vi "PLC_comm.vi"() -> ()   [LabVIEW 2017]
uses:
  <vilib>/DATA AHEAD/SP7/typedefs/PLC Type.ctl
  <vilib>/Utility/error.llb/DialogType.ctl
  <vilib>/addons/database/Connection.llb/DB Tools Open Connec (String).vi
  Global/Global 1.vi
  Global/DATA LOG.vi
  <vilib>/DATA AHEAD/SP7/functions/write/write Dint array.vi
  <vilib>/DATA AHEAD/SP7/functions/write/writeString.vi
  <vilib>/DATA AHEAD/SP7/functions/read/read Dint array.vi
  <vilib>/DATA AHEAD/SP7/functions/read/read real array.vi
  <vilib>/DATA AHEAD/SP7/functions/read/read String.vi
  <vilib>/addons/database/NI_Database_API.lvlib
  <vilib>/DATA AHEAD/SP7/SP7.lvlib
panel:
  out "IP1 7":string
  out "PLC 7":bool
  out "IP1 6":string
  out "PLC 6":bool
  out "IP1 5":string
  out "PLC 5":bool
  out "PLC 4":bool
  out "PLC 3":bool
  out "PLC 2":bool
  out "PLC 1":bool
  out "IP1 4":string
  out "IP1 3":string
  out "IP1 2":string
  out "IP1":string
  in  "stop":bool
  out "error out":errorcluster
  in  "error in (no error)":errorcluster
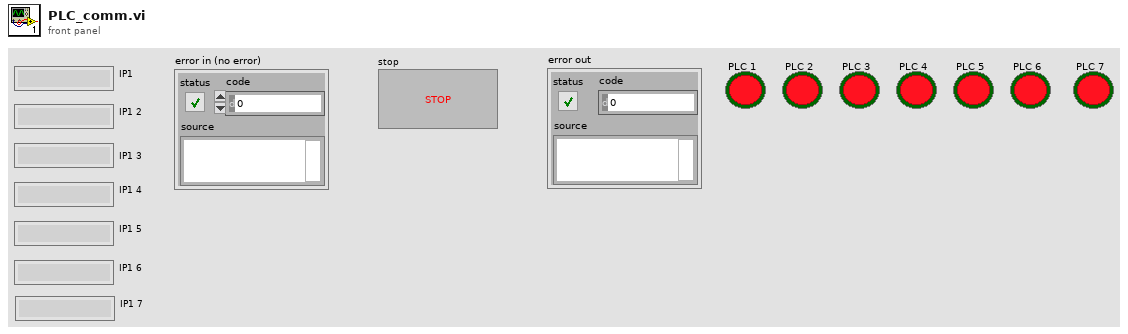
[diagram p1: front panel]
types:
  T1 = typedef "DialogType.ctl" = u16
  T2 = typedef "SP7.lvlib/PLC Type.ctl" = enum16{"S7 200", "S7 300/400", "S7 1200", "S7 1500", "LOGO!8"}
  T3 = typedef "NI_Database_API.lvlib/Conn ObjectReference.ctl" = refnum<k1>
  T4 = typedef "SP7.lvlib/S7 Connection.ctl" = cluster{"TCP Connection Ref":refnum<k5>, "IP address":string, "timeout ms":i32, "Connected?":bool, "PLC Type":T2, "Rack S7 400":u8, "Slot S7 400":u8, "PDU Size":u16, "connection semaphore":T5}
  T5 = typedef "Semaphore RefNum" = refnum<k1>
diagram:
  w2 = T1 0 items=["no dialog", "OK message", "continue or stop message", "OK message + warnings", "continue/stop + warnings"]  # type of dialog (OK msg:1)
  w4 = i32[] [0, 0, 0, 0, 0]  # I/P
  w5 = i32[] [0, 0]  # Input
  w7 = i32[] [0, 0]  # Input
  w8 = i32[] [0, 0]  # Input
  w10 = i32[] [0, 0]  # Input
  w6 = i32[] [0, 0, 0, 0, 0]  # I/P
  w9 = i32[] [0, 0, 0, 0, 0]  # I/P
  w11 = i32[] [0, 0, 0, 0, 0]  # I/P
  w12 = i32[] [0, 0, 0, 0, 0]  # I/P
  w13 = i32[] [0, 0]  # Input
  w14 = i32[] [0, 0]  # Input
  w15 = i32[] [0, 0, 0, 0, 0]  # I/P
  w16 = i32[] [0, 0, 0, 0, 0]  # I/P
  w17 = i32[] [0, 0]  # Input
  w18 = i32[] [0, 0]  # I/P
  w19 = i32[] [0, 0]  # Input
  # "OP 80"
  # "OP 70"
  # "OP 60"
  # "OP 50"
  # "OP 40"
  # "OP 30"
  # "OP 20"
  # "OP 10"
  n1 = call "path_db.vi"("error in"="error in (no error)") -> ("error out"=w171:errorcluster, "resulting string"=w176:string)  [unwired: 9 in]
  n2 = call-poly <vilib>:"DB Tools Open Connection.vi"("error in (no error)"=w171, "connection information"=w176) -> ("error out"=w175:errorcluster, "connection reference"=w174:T3)  [unwired: 6 in]
  n3 = call <vilib>:"DB Tools Select Data.vi"("error in (no error)"=w175, "columns"=string[] ["PLC_IP_1", "PLC_IP_2", "PLC_IP_3", "PLC_IP_4", "PLC_IP_5", "PLC_IP_6", "PLC_IP_7"], "table"="IP_SETTING", "connection reference"=w174) -> ("error out"=w173:errorcluster, "data"=w172:variant[][])  [unwired: 2 in, 1 out]
  n4 = call "PADMINI_varient_to_data.vi"("error in (no error)"=w173, "data"=w172) -> ("error out"=w26:errorcluster, "Array"=w167:string[][])  [unwired: 8 in]
  n5 = call "PADMINI_AUTO_CYCLE STATE.vi"("Enum"=enum16{"Read", "Write"}."Write", "error in (no error)"=w26, "Input"=w19) -> ("error out"=w153:errorcluster)  [unwired: 7 in, 1 out]
  n6 = Index Array(array=w167, index (row)=0) -> (element=w166:string[])  [unwired: 1 in]
  n7 = call "PADMINI_AUTO_BARCODE_STRING.vi"("Enum"=enum16{"Read", "Write"}."Write", "error in (no error)"=w153, "Input"=string[] ["", ""]) -> ("error out"=w150:errorcluster)  [unwired: 7 in, 1 out]
  n8 = call "PADMINI_AUTO_BARCODE_STATUS.vi"("Enum"=enum16{"Read", "Write"}."Write", "error in (no error)"=w150, "I/P"=w18) -> ("error out"=w148:errorcluster)  [unwired: 7 in, 1 out]
  n9 = call "PADMINI_AUTO_CYCLE VALUE 10.vi"("Enum"=enum16{"Read", "Write"}."Write", "error in (no error)"=w148, "Input"=dbl[] [0.0]) -> ("error out"=w142:errorcluster)  [unwired: 7 in, 1 out]
  n10 = call "PADMINI_AUTO_CYCLE STATE 20.vi"("Enum"=enum16{"Read", "Write"}."Write", "error in (no error)"=w142, "Input"=w5) -> ("error out"=w140:errorcluster)  [unwired: 7 in, 1 out]
  n11 = call "PADMINI_AUTO_CYCLE VALUE 20.vi"("Enum"=enum16{"Read", "Write"}."Write", "error in (no error)"=w140, "Input"=dbl[] [0.0, 0.0, 0.0, 0.0]) -> ("error out"=w136:errorcluster)  [unwired: 7 in, 1 out]
  n12 = call "PADMINI_AUTO_BARCODE_STRING2.vi"("Enum"=enum16{"Read", "Write"}."Write", "error in (no error)"=w136, "Input"=string[] ["", "", "", "", "", "", ""]) -> ("error out"=w134:errorcluster)  [unwired: 7 in, 1 out]
  n13 = call "PADMINI_AUTO_BARCODE_STATUS 20.vi"("Enum"=enum16{"Read", "Write"}."Write", "error in (no error)"=w134, "I/P"=w4) -> ("error out"=w128:errorcluster)  [unwired: 7 in, 1 out]
  n14 = call "PADMINI_AUTO_BARCODE_STATUS 30.vi"("Enum"=enum16{"Read", "Write"}."Write", "error in (no error)"=w128, "I/P"=w6) -> ("error out"=w125:errorcluster)  [unwired: 7 in, 1 out]
  n15 = call "PADMINI_AUTO_CYCLE STATE 30.vi"("Enum"=enum16{"Read", "Write"}."Write", "error in (no error)"=w125, "Input"=w7) -> ("error out"=w124:errorcluster)  [unwired: 7 in, 1 out]
  n16 = call "PADMINI_AUTO_CYCLE VALUE 30.vi"("Enum"=enum16{"Read", "Write"}."Write", "error in (no error)"=w124, "Input"=dbl[] [0.0, 0.0]) -> ("error out"=w121:errorcluster)  [unwired: 7 in, 1 out]
  n17 = call "PADMINI_AUTO_BARCODE_STRING 30.vi"("Enum"=enum16{"Read", "Write"}."Write", "error in (no error)"=w121, "Input"=string[] ["", "", ""]) -> ("error out"=w100:errorcluster)  [unwired: 7 in, 1 out]
  n18 = call "PADMINI_AUTO_BARCODE_STATUS 40.vi"("Enum"=enum16{"Read", "Write"}."Write", "error in (no error)"=w100, "I/P"=w9) -> ("error out"=w99:errorcluster)  [unwired: 7 in, 1 out]
  n19 = call "PADMINI_AUTO_CYCLE VALUE 40.vi"("Enum"=enum16{"Read", "Write"}."Write", "error in (no error)"=w99, "Input"=dbl[] [0.0, 0.0, 0.0, 0.0]) -> ("error out"=w98:errorcluster)  [unwired: 7 in, 1 out]
  n20 = call "PADMINI_AUTO_CYCLE STATE 40.vi"("Enum"=enum16{"Read", "Write"}."Write", "error in (no error)"=w98, "Input"=w8) -> ("error out"=w97:errorcluster)  [unwired: 7 in, 1 out]
  n21 = call "PADMINI_AUTO_BARCODE_STATUS 50.vi"("Enum"=enum16{"Read", "Write"}."Write", "error in (no error)"=w97, "I/P"=w11) -> ("error out"=w82:errorcluster)  [unwired: 7 in, 1 out]
  n22 = call "PADMINI_AUTO_CYCLE STATE 50.vi"("Enum"=enum16{"Read", "Write"}."Write", "error in (no error)"=w82, "Input"=w10) -> ("error out"=w86:errorcluster)  [unwired: 7 in, 1 out]
  n23 = call "PADMINI_AUTO_CYCLE VALUE 50.vi"("Enum"=enum16{"Read", "Write"}."Write", "error in (no error)"=w86, "Input"=dbl[] [0.0, 0.0, 0.0]) -> ("error out"=w83:errorcluster)  [unwired: 7 in, 1 out]
  n24 = call "PADMINI_AUTO_BARCODE_STRING 50.vi"("Enum"=enum16{"Read", "Write"}."Write", "error in (no error)"=w83, "Input"=string[] ["", "", "", "", "", ""]) -> ("error out"=w59:errorcluster)  [unwired: 7 in, 1 out]
  n25 = call "PADMINI_AUTO_BARCODE_STATUS 60.vi"("Enum"=enum16{"Read", "Write"}."Write", "error in (no error)"=w59, "I/P"=w12) -> ("error out"=w63:errorcluster)  [unwired: 7 in, 1 out]
  n26 = call "PADMINI_AUTO_CYCLE STATE 60.vi"("Enum"=enum16{"Read", "Write"}."Write", "error in (no error)"=w63, "Input"=w13) -> ("error out"=w65:errorcluster)  [unwired: 7 in, 1 out]
  n27 = call "PADMINI_AUTO_CYCLE VALUE 60.vi"("Enum"=enum16{"Read", "Write"}."Write", "error in (no error)"=w65, "Input"=dbl[] [0.0, 0.0, 0.0, 0.0, 0.0]) -> ("error out"=w68:errorcluster)  [unwired: 7 in, 1 out]
  n28 = call "PADMINI_AUTO_BARCODE_STRING 60.vi"("Enum"=enum16{"Read", "Write"}."Write", "error in (no error)"=w68, "Input"=string[] ["", "", "", "", "", ""]) -> ("error out"=w35:errorcluster)  [unwired: 7 in, 1 out]
  n29 = call "PADMINI_AUTO_BARCODE_STATUS 70.vi"("Enum"=enum16{"Read", "Write"}."Write", "error in (no error)"=w35, "I/P"=w15) -> ("error out"=w38:errorcluster)  [unwired: 7 in, 1 out]
  n30 = call "PADMINI_AUTO_CYCLE STATE 70.vi"("Enum"=enum16{"Read", "Write"}."Read", "error in (no error)"=w38, "Input"=w14) -> ("error out"=w50:errorcluster)  [unwired: 7 in, 1 out]
  n31 = call "PADMINI_AUTO_CYCLE VALUE 70.vi"("Enum"=enum16{"Read", "Write"}."Write", "error in (no error)"=w50, "Input"=dbl[] [0.0, 0.0]) -> ("error out"=w47:errorcluster)  [unwired: 7 in, 1 out]
  n32 = call "PADMINI_AUTO_BARCODE_STRING 70.vi"("Enum"=enum16{"Read", "Write"}."Write", "error in (no error)"=w47, "Input"=string[] ["", ""]) -> ("error out"=w32:errorcluster)  [unwired: 7 in, 1 out]
  n33 = call "PADMINI_AUTO_BARCODE_STATUS 80.vi"("Enum"=enum16{"Read", "Write"}."Write", "error in (no error)"=w32, "I/P"=w16) -> ("error out"=w39:errorcluster)  [unwired: 7 in, 1 out]
  n34 = call "PADMINI_AUTO_CYCLE STATE 80.vi"("Enum"=enum16{"Read", "Write"}."Write", "error in (no error)"=w39, "Input"=w17) -> ("error out"=w43:errorcluster)  [unwired: 7 in, 1 out]
  n35 = call "PADMINI_AUTO_CYCLE VALUE 80.vi"("Enum"=enum16{"Read", "Write"}."Write", "error in (no error)"=w43, "Input"=sgl[] [0.0]) -> ("error out"=w46:errorcluster)  [unwired: 7 in, 1 out]
  n36 = call "PADMINI_AUTO_BARCODE_STRING 80.vi"("Enum"=enum16{"Read", "Write"}."Write", "error in (no error)"=w46, "Input"=string[] ["", "", ""]) -> ()  [unwired: 7 in, 2 out]
  n37 = Index Array(array=w166) -> (element #1=w115:string, element #2=w116:string, element #3=w110:string, element #4=w88:string, element #5=w71:string, element #6=w28:string, element #7=w27:string)  [unwired: 7 in]
  "IP1" <- w115
  "IP1 2" <- w116
  "IP1 3" <- w110
  "IP1 4" <- w88
  "IP1 5" <- w71
  "IP1 6" <- w28
  "IP1 7" <- w27
  n38 = call <vilib>:"connect.vi"("PLC Type"=PLC_Type."S7 1200" ("PLC Type 2"), "error in (no error)"=w26, "timeout [ms]"=1000 ("timeout [ms] 2"), "IP address"=w27) -> ("error out"=w29:errorcluster, "S7 Connection out"=w1:T4)  [unwired: 6 in]
  n39 = call <vilib>:"connect.vi"("PLC Type"=PLC_Type."S7 1200" ("PLC Type 2"), "error in (no error)"=w26, "timeout [ms]"=1000 ("timeout [ms] 2"), "IP address"=w71) -> ("error out"=w76:errorcluster, "S7 Connection out"=w75:T4)  [unwired: 6 in]
  n40 = call <vilib>:"connect.vi"("PLC Type"=PLC_Type."S7 1200" ("PLC Type 2"), "error in (no error)"=w26, "timeout [ms]"=1000 ("timeout [ms] 2"), "IP address"=w28) -> ("error out"=w56:errorcluster, "S7 Connection out"=w55:T4)  [unwired: 6 in]
  n41 = call <vilib>:"connect.vi"("PLC Type"=PLC_Type."S7 1200" ("PLC Type 2"), "error in (no error)"=w26, "timeout [ms]"=1000 ("timeout [ms] 2"), "IP address"=w88) -> ("error out"=w91:errorcluster, "S7 Connection out"=w92:T4)  [unwired: 6 in]
  n42 = call <vilib>:"connect.vi"("PLC Type"=PLC_Type."S7 1200" ("PLC Type 2"), "error in (no error)"=w26, "timeout [ms]"=1000 ("timeout [ms] 2"), "IP address"=w116) -> ("error out"=w131:errorcluster, "S7 Connection out"=w130:T4)  [unwired: 6 in]
  n43 = call <vilib>:"connect.vi"("PLC Type"=PLC_Type."S7 1200" ("PLC Type 2"), "error in (no error)"=w26, "timeout [ms]"=1000 ("timeout [ms] 2"), "IP address"=w110) -> ("error out"=w112:errorcluster, "S7 Connection out"=w111:T4)  [unwired: 6 in]
  n44 = call <vilib>:"connect.vi"("PLC Type"=PLC_Type."S7 1200" ("PLC Type 2"), "error in (no error)"=w26, "timeout [ms]"=1000, "IP address"=w115) -> ("error out"=w157:errorcluster, "S7 Connection out"=w156:T4)  [unwired: 6 in]
  n45 = while {
    shift-right: [w179] -> w23
    shift-left: w1 -> [w189]
    shift-right: [w187] -> w24
    shift-left: w29 -> [w188]
    tunnel: w27 -> [w178]
    stop <- w181 stop-if-true
    # "OP 90 - 100 - 110"
    n46 = flat-sequence {
      tunnel: [w265] -> w185
      tunnel: [w266] -> w180
      tunnel: w188 -> [w304]
      tunnel: w189 -> [w303]
      tunnel: w178 -> [w285]
      tunnel: [w285] -> w177
      tunnel: [w372] -> w187
      tunnel: [w371] -> w179
      tunnel: w185 -> [w374]
      tunnel: w180 -> [w373]
      tunnel: w177 -> [w370]
      frame #0 {
        w206 = u16 75 ("Data Block #")
        w231 = u16 72 ("Data Block #")
        w257 = u16 70 ("Data Block #")
        w215 = u16 71 ("Data Block #")
        w245 = u16 69 ("Data Block #")
        # "OP100 OK\nOP 100 NG"
        # "AUTO WRITE"
        n47 = global read "DATA LOG.vi" "OP 90 Outputs"() -> (w302:bool)
        n48 = case shown="True" w302 {
          tunnel: w303 -> [w355 w368]
          tunnel: [w356 w357] -> w262
          tunnel: [w355 w358] -> w263
          tunnel: w304 -> [w356 w365]
          frame False {
          }
          frame True {
            w369 = u16 70  # Data Block #
            n49 = call "PADMINI_AUTO_BARCODE_STATUS 90.vi"("Enum"=enum16{"Read", "Write"}."Read", "error in (no error)"=w365) -> ("error out"=w364:errorcluster, "O/P"=w366:i32[])  [unwired: 8 in]
            n50 = global write "DATA LOG.vi" "OP 90 Outputs"(FALSE) -> ()
            n51 = call-poly <vilib>:"write DB.vi"("DINT input array"=w366, "error in (no error)"=w364, "Data Block #"=w369, "S7 Connection in"=w368) -> ("error out"=w360:errorcluster, "S7 Connection out"=w359:T4)  [unwired: 4 in, 2 out]
            n52 = call-poly <vilib>:"write DB.vi"("DINT input array"=i32[] [0] ("Data Byte"), "error in (no error)"=w360, "Data Block #"=u16 69, "S7 Connection in"=w359) -> ("error out"=w357:errorcluster, "S7 Connection out"=w358:T4)  [unwired: 4 in, 2 out]
          }
        }
        n53 = global read "DATA LOG.vi" "OP 90 reset"() -> (w261:bool)
        n54 = case shown="True" w261 {
          tunnel: w262 -> [w330 w339]
          tunnel: [w330 w338] -> w250
          tunnel: w263 -> [w331 w337]
          tunnel: [w331 w336] -> w251
          frame False {
          }
          frame True {
            n55 = global write "DATA LOG.vi" "OP 90 reset"(FALSE) -> ()
            n56 = call-poly <vilib>:"write DB.vi"("Item offset [byte]"=u16 4 ("Data Block #"), "DINT input array"=i32[] [0], "error in (no error)"=w339, "Data Block #"=u16 69, "S7 Connection in"=w337) -> ("error out"=w338:errorcluster, "S7 Connection out"=w336:T4)  [unwired: 3 in, 2 out]
          }
        }
        n57 = global read "DATA LOG.vi" "Auto Cycle On"() -> (w197:bool)
        n58 = Boolean To (0,1)(Boolean=w197) -> (0, 1=w196:i16)
        n59 = Build Array(w196) -> (w195:i16[])
        n60 = global read "Global 1.vi" "Filtered BARCODE selected"() -> (w260:string[])
        n61 = call-poly <vilib>:"write DB.vi"("Item offset [byte]"=u32 20, "DINT input array"=w195, "error in (no error)"=w250, "Data Block #"=w257, "S7 Connection in"=w251) -> ("error out"=w255:errorcluster, "S7 Connection out"=w254:T4)  [unwired: 3 in, 2 out]
        n62 = call-poly <vilib>:"write DB.vi"("Item offset [byte]"=u32 24, "Input STRINGS"=w260, "error in (no error)"=w255, "String length reserved in DB (default=254)"=u16 15, "Data Block #"=w257, "S7 Connection in"=w254) -> ("error out"=w252:errorcluster, "S7 Connection out"=w253:T4)  [unwired: 2 in, 2 out]
        n63 = call-poly <vilib>:"read DB.vi"("error in (no error)"=w252, "items #"=u16 2 ("Items # [byte]"), "Data Block #"=w245, "S7 Connection in"=w253) -> ("error out"=w300:errorcluster, "DINT result array"=w298:i32[], "S7 Connection out"=w295:T4)  [unwired: 5 in]
        n64 = call "PADMINI_AUTO_CYCLE STATE 90.vi"("Enum"=enum16{"Read", "Write"}."Write", "error in (no error)"=w300, "Input"=w298) -> ("error out"=w296:errorcluster)  [unwired: 7 in, 1 out]
        n65 = call-poly <vilib>:"read DB.vi"("Item offset [byte]"=u32 8, "error in (no error)"=w296, "items #"=u16 2 ("Items # [byte]"), "Data Block #"=w245, "S7 Connection in"=w295) -> ("error out"=w288:errorcluster, "REAL result array"=w286:sgl[], "S7 Connection out"=w294:T4)  [unwired: 4 in]
        n66 = call "PADMINI_AUTO_CYCLE VALUE 90.vi"("Enum"=enum16{"Read", "Write"}."Write", "error in (no error)"=w288, "Input"=w286) -> ("error out"=w287:errorcluster)  [unwired: 7 in, 1 out]
        n67 = call-poly <vilib>:"read DB.vi"("Item offset [byte]"=u32 16, "String length reserved in DB (default=254)"=u16 50, "error in (no error)"=w287, "items #"=u16 1 ("Items # [byte]"), "Data Block #"=w245, "S7 Connection in"=w294) -> ("error out"=w249:errorcluster, "STRING result Array"=w240:string[], "S7 Connection out"=w248:T4)  [unwired: 2 in, 1 out]
        n68 = call-poly <vilib>:"read DB.vi"("Item offset [byte]"=u32 68, "String length reserved in DB (default=254)"=u16 10, "error in (no error)"=w249, "items #"=u16 3 ("Items # [byte]"), "Data Block #"=w245, "S7 Connection in"=w248) -> ("error out"=w247:errorcluster, "STRING result Array"=w239:string[], "S7 Connection out"=w246:T4)  [unwired: 2 in, 1 out]
        n69 = Build Array (concatenate)(w240, w239) -> (w238:string[])
        n70 = call "PADMINI_AUTO_BARCODE_STRING 90.vi"("Enum"=enum16{"Read", "Write"}."Write", "error in (no error)"=w247, "Input"=w238) -> ("error out"=w267:errorcluster)  [unwired: 7 in, 1 out]
        n71 = global read "DATA LOG.vi" "OP 100 Outputs"() -> (w268:bool)
        n72 = case shown="True" w268 {
          tunnel: w246 -> [w340 w353]
          tunnel: [w341 w344] -> w236
          tunnel: [w340 w345] -> w237
          tunnel: w267 -> [w341 w350]
          frame False {
          }
          frame True {
            w354 = u16 72  # Data Block #
            n73 = call "PADMINI_AUTO_BARCODE_STATUS 100.vi"("Enum"=enum16{"Read", "Write"}."Read", "error in (no error)"=w350) -> ("error out"=w349:errorcluster, "O/P"=w351:i32[])  [unwired: 8 in]
            n74 = global write "DATA LOG.vi" "OP 100 Outputs"(FALSE) -> ()
            n75 = call-poly <vilib>:"write DB.vi"("DINT input array"=w351, "error in (no error)"=w349, "Data Block #"=w354, "S7 Connection in"=w353) -> ("error out"=w343:errorcluster, "S7 Connection out"=w342:T4)  [unwired: 4 in, 2 out]
            n76 = call-poly <vilib>:"write DB.vi"("DINT input array"=i32[] [0] ("Data Byte"), "error in (no error)"=w343, "Data Block #"=u16 71, "S7 Connection in"=w342) -> ("error out"=w344:errorcluster, "S7 Connection out"=w345:T4)  [unwired: 4 in, 2 out]
          }
        }
        n77 = global read "DATA LOG.vi" "OP 100 reset"() -> (w235:bool)
        n78 = case shown="True" w235 {
          tunnel: w236 -> [w320 w329]
          tunnel: [w320 w328] -> w227
          tunnel: w237 -> [w321 w327]
          tunnel: [w321 w326] -> w226
          frame False {
          }
          frame True {
            n79 = global write "DATA LOG.vi" "OP 100 reset"(FALSE) -> ()
            n80 = call-poly <vilib>:"write DB.vi"("Item offset [byte]"=u16 4 ("Data Block #"), "DINT input array"=i32[] [0], "error in (no error)"=w329, "Data Block #"=u16 71, "S7 Connection in"=w327) -> ("error out"=w328:errorcluster, "S7 Connection out"=w326:T4)  [unwired: 3 in, 2 out]
          }
        }
        n81 = global read "DATA LOG.vi" "Auto Cycle On"() -> (w194:bool)
        n82 = Boolean To (0,1)(Boolean=w194) -> (0, 1=w193:i16)
        n83 = Build Array(w193) -> (w192:i16[])
        n84 = global read "Global 1.vi" "Filtered BARCODE selected"() -> (w228:string[])
        n85 = call-poly <vilib>:"write DB.vi"("Item offset [byte]"=u32 20, "DINT input array"=w192, "error in (no error)"=w227, "Data Block #"=w231, "S7 Connection in"=w226) -> ("error out"=w233:errorcluster, "S7 Connection out"=w234:T4)  [unwired: 3 in, 2 out]
        n86 = call-poly <vilib>:"write DB.vi"("Item offset [byte]"=u32 24, "Input STRINGS"=w228, "error in (no error)"=w233, "String length reserved in DB (default=254)"=u16 15, "Data Block #"=w231, "S7 Connection in"=w234) -> ("error out"=w224:errorcluster, "S7 Connection out"=w225:T4)  [unwired: 2 in, 2 out]
        n87 = call-poly <vilib>:"read DB.vi"("error in (no error)"=w224, "items #"=u16 2 ("Items # [byte]"), "Data Block #"=w215, "S7 Connection in"=w225) -> ("error out"=w270:errorcluster, "DINT result array"=w272:i32[], "S7 Connection out"=w275:T4)  [unwired: 5 in]
        n88 = call "PADMINI_AUTO_CYCLE STATE 100.vi"("Enum"=enum16{"Read", "Write"}."Write", "error in (no error)"=w270, "Input"=w272) -> ("error out"=w274:errorcluster)  [unwired: 7 in, 1 out]
        n89 = call-poly <vilib>:"read DB.vi"("Item offset [byte]"=u32 8, "error in (no error)"=w274, "items #"=u16 11 ("Items # [byte]"), "Data Block #"=w215, "S7 Connection in"=w275) -> ("error out"=w282:errorcluster, "REAL result array"=w284:sgl[], "S7 Connection out"=w276:T4)  [unwired: 4 in]
        n90 = call "PADMINI_AUTO_CYCLE VALUE 100.vi"("Enum"=enum16{"Read", "Write"}."Write", "error in (no error)"=w282, "Input"=w284) -> ("error out"=w283:errorcluster)  [unwired: 7 in, 1 out]
        n91 = call-poly <vilib>:"read DB.vi"("Item offset [byte]"=u32 52, "String length reserved in DB (default=254)"=u16 50, "error in (no error)"=w283, "items #"=u16 1 ("Items # [byte]"), "Data Block #"=w215, "S7 Connection in"=w276) -> ("error out"=w221:errorcluster, "STRING result Array"=w218:string[], "S7 Connection out"=w220:T4)  [unwired: 2 in, 1 out]
        n92 = call-poly <vilib>:"read DB.vi"("Item offset [byte]"=u32 104, "String length reserved in DB (default=254)"=u16 10, "error in (no error)"=w221, "items #"=u16 2 ("Items # [byte]"), "Data Block #"=w215, "S7 Connection in"=w220) -> ("error out"=w222:errorcluster, "STRING result Array"=w216:string[], "S7 Connection out"=w219:T4)  [unwired: 2 in, 1 out]
        n93 = Build Array (concatenate)(w218, w216) -> (w217:string[])
        n94 = call "PADMINI_AUTO_BARCODE_STRING 100.vi"("Enum"=enum16{"Read", "Write"}."Write", "error in (no error)"=w222, "Input"=w217) -> ("error out"=w264:errorcluster)  [unwired: 7 in, 1 out]
        n95 = global read "DATA LOG.vi" "OP 110 Outputs"() -> (w212:bool)
        n96 = case shown="True" w212 {
          tunnel: [w305 w310] -> w198
          tunnel: [w306 w311] -> w199
          tunnel: w264 -> [w305 w315]
          tunnel: w219 -> [w306 w314]
          frame False {
          }
          frame True {
            w307 = i32[] [0]  # DINT input array
            w308 = u16 75  # Data Block #
            n97 = call "PADMINI_AUTO_BARCODE_STATUS 110.vi"("Enum"=enum16{"Read", "Write"}."Read", "error in (no error)"=w315) -> ("error out"=w317:errorcluster, "O/P"=w318:i32[])  [unwired: 8 in]
            n98 = call-poly <vilib>:"write DB.vi"("Item offset [byte]"=u32 4, "DINT input array"=w318, "error in (no error)"=w317, "Data Block #"=w308, "S7 Connection in"=w314) -> ("error out"=w309:errorcluster, "S7 Connection out"=w312:T4)  [unwired: 3 in, 2 out]
            n99 = global write "DATA LOG.vi" "OP 110 Outputs"(FALSE) -> ()
            n100 = call-poly <vilib>:"write DB.vi"("DINT input array"=w307, "error in (no error)"=w309, "Data Block #"=w308, "S7 Connection in"=w312) -> ("error out"=w310:errorcluster, "S7 Connection out"=w311:T4)  [unwired: 4 in, 2 out]
          }
        }
        n101 = call-poly <vilib>:"read DB.vi"("error in (no error)"=w198, "items #"=u16 1 ("Items # [byte]"), "Data Block #"=w206, "S7 Connection in"=w199) -> ("error out"=w210:errorcluster, "DINT result array"=w208:i32[], "S7 Connection out"=w207:T4)  [unwired: 5 in]
        n102 = call "PADMINI_AUTO_CYCLE STATE 110.vi"("Enum"=enum16{"Read", "Write"}."Write", "error in (no error)"=w210, "Input"=w208) -> ("error out"=w200:errorcluster)  [unwired: 7 in, 1 out]
        n103 = call-poly <vilib>:"read DB.vi"("Item offset [byte]"=u32 12, "String length reserved in DB (default=254)"=u16 50, "error in (no error)"=w200, "items #"=u16 1 ("Items # [byte]"), "Data Block #"=w206, "S7 Connection in"=w207) -> ("error out"=w202:errorcluster, "STRING result Array"=w203:string[], "S7 Connection out"=w265:T4)  [unwired: 2 in, 1 out]
        n104 = call "PADMINI_AUTO_BARCODE_STRING 110.vi"("Enum"=enum16{"Read", "Write"}."Write", "error in (no error)"=w202, "Input"=w203) -> ("error out"=w266:errorcluster)  [unwired: 7 in, 1 out]
      }
      frame #1 {
        # "RECONNECT"
        n105 = case shown="Error" w373 {
          selector: w373 -> [w378 w386]
          tunnel: [w377 w383] -> w371
          tunnel: [w378 w384] -> w372
          tunnel: w374 -> [w377 w380]
          tunnel: w370 -> [_ w379]
          frame No Error {
          }
          frame Error {
            n106 = call <vilib>:"Clear Errors.vi"("error in (no error)"=w386) -> ("error out"=w387:errorcluster)  [unwired: 5 in, 1 out]
            n107 = call <vilib>:"disconnect.vi"("error in (no error)"=w387, "S7 Connection in"=w380) -> ("error out"=w385:errorcluster)  [unwired: 8 in, 1 out]
            n108 = call <vilib>:"Clear Errors.vi"("error in (no error)"=w385) -> ("error out"=w382:errorcluster)  [unwired: 5 in, 1 out]
            n109 = call <vilib>:"connect.vi"("PLC Type"=PLC_Type."S7 1200" ("PLC Type 2"), "error in (no error)"=w382, "IP address"=w379) -> ("error out"=w384:errorcluster, "S7 Connection out"=w383:T4)  [unwired: 7 in]
          }
        }
        n110 = Unbundle By Name(w373) -> ("status"=w376:bool)
        n111 = Not(x=w376) -> (.not. x?=w375:bool)
        "PLC 7" <- w375
        n112 = global write "Global 1.vi" "PLC 7"(w375) -> ()
      }
    }
    n113 = call "PADMINI_STOP_ALL.vi"("Enum"=enum16{"Read", "Write"}."Read") -> ("Boolean 2"=w183:bool)  [unwired: 9 in, 1 out]
    n114 = local read "stop"() -> (w182:bool)
    n115 = Or(x=w182, y=w183) -> (x .or. y?=w181:bool)
    n116 = Wait (ms)(milliseconds to wait=u32 50) -> ()  [unwired: 1 out]
  }
  n117 = while {
    shift-right: [w390] -> w118
    shift-left: w130 -> [w400]
    shift-right: [w398] -> w117
    shift-left: w131 -> [w399]
    tunnel: w116 -> [w389]
    stop <- w392 stop-if-true
    # "OP 30"
    n118 = flat-sequence {
      tunnel: [w403] -> w396
      tunnel: [w405] -> w391
      tunnel: w399 -> [w407]
      tunnel: w400 -> [w406]
      tunnel: w389 -> [w404]
      tunnel: [w404] -> w388
      tunnel: [w410] -> w398
      tunnel: [w409] -> w390
      tunnel: w396 -> [w412]
      tunnel: w391 -> [w411]
      tunnel: w388 -> [w408]
      frame #0 {
        # "AUTO WRITE"
        n119 = call "PLC_OP30_Write.vi"("error in (no error)"=w407, "S7 Connection in"=w406) -> ("error out"=w401:errorcluster, "S7 Connection out"=w402:T4)  [unwired: 8 in]
        n120 = call "PLC_OP30_Read.vi"("error in (no error)"=w401, "S7 Connection in"=w402) -> ("error out"=w405:errorcluster, "S7 Connection out 2"=w403:T4)  [unwired: 8 in]
      }
      frame #1 {
        # "RECONNECT"
        n121 = case shown="Error" w411 {
          selector: w411 -> [w416 w424]
          tunnel: [w415 w421] -> w409
          tunnel: [w416 w422] -> w410
          tunnel: w412 -> [w415 w418]
          tunnel: w408 -> [_ w417]
          frame No Error {
          }
          frame Error {
            n122 = call <vilib>:"Clear Errors.vi"("error in (no error)"=w424) -> ("error out"=w425:errorcluster)  [unwired: 5 in, 1 out]
            n123 = call <vilib>:"disconnect.vi"("error in (no error)"=w425, "S7 Connection in"=w418) -> ("error out"=w423:errorcluster)  [unwired: 8 in, 1 out]
            n124 = call <vilib>:"Clear Errors.vi"("error in (no error)"=w423) -> ("error out"=w420:errorcluster)  [unwired: 5 in, 1 out]
            n125 = call <vilib>:"connect.vi"("PLC Type"=PLC_Type."S7 1200" ("PLC Type 2"), "error in (no error)"=w420, "IP address"=w417) -> ("error out"=w422:errorcluster, "S7 Connection out"=w421:T4)  [unwired: 7 in]
          }
        }
        n126 = Unbundle By Name(w411) -> ("status"=w414:bool)
        n127 = Not(x=w414) -> (.not. x?=w413:bool)
        "PLC 2" <- w413
        n128 = global write "Global 1.vi" "PLC 2"(w413) -> ()
      }
    }
    n129 = call "PADMINI_STOP_ALL.vi"("Enum"=enum16{"Read", "Write"}."Read") -> ("Boolean 2"=w394:bool)  [unwired: 9 in, 1 out]
    n130 = Wait (ms)(milliseconds to wait=u32 50) -> ()  [unwired: 1 out]
    n131 = local read "stop"() -> (w393:bool)
    n132 = Or(x=w393, y=w394) -> (x .or. y?=w392:bool)
  }
  n133 = while {
    shift-right: [w428] -> w145
    shift-left: w156 -> [w438]
    shift-right: [w436] -> w160
    shift-left: w157 -> [w437]
    tunnel: w115 -> [w426]
    stop <- w431 stop-if-true
    # "OP 10 AND 20"
    n134 = flat-sequence {
      tunnel: [w441] -> w430
      tunnel: [w447] -> w429
      tunnel: w437 -> [w448]
      tunnel: w438 -> [w449]
      tunnel: [w446] -> w427
      tunnel: w426 -> [w446]
      tunnel: [w453] -> w436
      tunnel: [w452] -> w428
      tunnel: w430 -> [w454]
      tunnel: w429 -> [w450]
      tunnel: w427 -> [w451]
      frame #0 {
        # "NEW CHANGES"
        n135 = call "PLC_OP10_Write.vi"("error in (no error)"=w448, "S7 Connection in"=w449) -> ("error out"=w444:errorcluster, "S7 Connection out"=w445:T4)  [unwired: 8 in]
        n136 = call "PLC_OP10_Read.vi"("error in (no error)"=w444, "S7 Connection in"=w445) -> ("error out"=w443:errorcluster, "S7 Connection out"=w442:T4)  [unwired: 8 in]
        n137 = call "PLC_OP20_Write.vi"("error in (no error)"=w443, "S7 Connection in"=w442) -> ("error out"=w439:errorcluster, "S7 Connection out"=w440:T4)  [unwired: 8 in]
        n138 = call "PLC_OP20_Read.vi"("error in (no error)"=w439, "S7 Connection in"=w440) -> ("error out"=w447:errorcluster, "S7 Connection out 2"=w441:T4)  [unwired: 8 in]
      }
      frame #1 {
        # "RECONNECT"
        n139 = Unbundle By Name(w450) -> ("status"=w456:bool)
        n140 = case shown="Error" w450 {
          selector: w450 -> [w458 w467]
          tunnel: [w457 w464] -> w452
          tunnel: [w458 w465] -> w453
          tunnel: w454 -> [w457 w461]
          tunnel: w451 -> [_ w460]
          frame No Error {
          }
          frame Error {
            w459 = 1000  # timeout [ms]
            n141 = call <vilib>:"Clear Errors.vi"("error in (no error)"=w467) -> ("error out"=w468:errorcluster)  [unwired: 5 in, 1 out]
            n142 = call <vilib>:"disconnect.vi"("error in (no error)"=w468, "S7 Connection in"=w461) -> ("error out"=w466:errorcluster)  [unwired: 8 in, 1 out]
            n143 = call <vilib>:"Clear Errors.vi"("error in (no error)"=w466) -> ("error out"=w463:errorcluster)  [unwired: 5 in, 1 out]
            n144 = call <vilib>:"connect.vi"("PLC Type"=PLC_Type."S7 1200" ("PLC Type 2"), "error in (no error)"=w463, "timeout [ms]"=w459, "IP address"=w460) -> ("error out"=w465:errorcluster, "S7 Connection out"=w464:T4)  [unwired: 6 in]
          }
        }
        n145 = Not(x=w456) -> (.not. x?=w455:bool)
        "PLC 1" <- w455
        n146 = global write "Global 1.vi" "PLC 1"(w455) -> ()
      }
    }
    n147 = call "PADMINI_STOP_ALL.vi"("Enum"=enum16{"Read", "Write"}."Read") -> ("Boolean 2"=w433:bool)  [unwired: 9 in, 1 out]
    n148 = Or(x="stop", y=w433) -> (x .or. y?=w431:bool)
    n149 = Wait (ms)(milliseconds to wait=u32 50) -> ()  [unwired: 1 out]
  }
  n150 = while {
    shift-right: [w471] -> w95
    shift-left: w92 -> [w481]
    shift-right: [w479] -> w94
    shift-left: w91 -> [w480]
    tunnel: w88 -> [w470]
    stop <- w473 stop-if-true
    # "OP 50"
    n151 = flat-sequence {
      tunnel: [w502] -> w477
      tunnel: [w512] -> w472
      tunnel: w480 -> [w531]
      tunnel: w481 -> [w530]
      tunnel: w470 -> [w511]
      tunnel: [w511] -> w469
      tunnel: [w559] -> w479
      tunnel: [w558] -> w471
      tunnel: w477 -> [w561]
      tunnel: w472 -> [w560]
      tunnel: w469 -> [w557]
      frame #0 {
        w493 = u16 57 ("Data Block #")
        w501 = u16 56 ("Data Block #")
        # "AUTO WRITE"
        n152 = global read "DATA LOG.vi" "OP 50 Outputs"() -> (w529:bool)
        n153 = case shown="True" w529 {
          tunnel: w530 -> [w542 w555]
          tunnel: [w543 w544] -> w510
          tunnel: [w542 w547] -> w509
          tunnel: w531 -> [w543 w552]
          frame False {
          }
          frame True {
            w556 = u16 57  # Data Block #
            n154 = call "PADMINI_AUTO_BARCODE_STATUS 50.vi"("Enum"=enum16{"Read", "Write"}."Read", "error in (no error)"=w552) -> ("error out"=w551:errorcluster, "O/P"=w553:i32[])  [unwired: 8 in]
            n155 = global write "DATA LOG.vi" "OP 50 Outputs"(FALSE) -> ()
            n156 = call-poly <vilib>:"write DB.vi"("DINT input array"=w553, "error in (no error)"=w551, "Data Block #"=w556, "S7 Connection in"=w555) -> ("error out"=w545:errorcluster, "S7 Connection out"=w546:T4)  [unwired: 4 in, 2 out]
            n157 = call-poly <vilib>:"write DB.vi"("DINT input array"=i32[] [0] ("Data Byte"), "error in (no error)"=w545, "Data Block #"=u16 56, "S7 Connection in"=w546) -> ("error out"=w544:errorcluster, "S7 Connection out"=w547:T4)  [unwired: 4 in, 2 out]
          }
        }
        n158 = global read "DATA LOG.vi" "OP 50 reset"() -> (w508:bool)
        n159 = global read "DATA LOG.vi" "Auto Cycle On"() -> (w484:bool)
        n160 = case shown="True" w508 {
          tunnel: w510 -> [w532 w541]
          tunnel: [w532 w540] -> w486
          tunnel: w509 -> [w533 w539]
          tunnel: [w533 w538] -> w489
          frame False {
          }
          frame True {
            n161 = global write "DATA LOG.vi" "OP 50 reset"(FALSE) -> ()
            n162 = call-poly <vilib>:"write DB.vi"("Item offset [byte]"=u16 4 ("Data Block #"), "DINT input array"=i32[] [0], "error in (no error)"=w541, "Data Block #"=u16 56, "S7 Connection in"=w539) -> ("error out"=w540:errorcluster, "S7 Connection out"=w538:T4)  [unwired: 3 in, 2 out]
          }
        }
        n163 = Boolean To (0,1)(Boolean=w484) -> (0, 1=w483:i16)
        n164 = Build Array(w483) -> (w482:i16[])
        n165 = global read "Global 1.vi" "Filtered BARCODE selected"() -> (w490:string[])
        n166 = call-poly <vilib>:"write DB.vi"("Item offset [byte]"=u32 20, "DINT input array"=w482, "error in (no error)"=w486, "Data Block #"=w493, "S7 Connection in"=w489) -> ("error out"=w495:errorcluster, "S7 Connection out"=w496:T4)  [unwired: 3 in, 2 out]
        n167 = call-poly <vilib>:"write DB.vi"("Item offset [byte]"=u32 24, "Input STRINGS"=w490, "error in (no error)"=w495, "String length reserved in DB (default=254)"=u16 15, "Data Block #"=w493, "S7 Connection in"=w496) -> ("error out"=w487:errorcluster, "S7 Connection out"=w488:T4)  [unwired: 2 in, 2 out]
        n168 = call-poly <vilib>:"read DB.vi"("error in (no error)"=w487, "items #"=u16 2 ("Items # [byte]"), "Data Block #"=w501, "S7 Connection in"=w488) -> ("error out"=w527:errorcluster, "DINT result array"=w525:i32[], "S7 Connection out"=w522:T4)  [unwired: 5 in]
        n169 = call "PADMINI_AUTO_CYCLE STATE 50.vi"("Enum"=enum16{"Read", "Write"}."Write", "error in (no error)"=w527, "Input"=w525) -> ("error out"=w523:errorcluster)  [unwired: 7 in, 1 out]
        n170 = call-poly <vilib>:"read DB.vi"("Item offset [byte]"=u32 8, "error in (no error)"=w523, "items #"=u16 3 ("Items # [byte]"), "Data Block #"=w501, "S7 Connection in"=w522) -> ("error out"=w515:errorcluster, "REAL result array"=w513:sgl[], "S7 Connection out"=w521:T4)  [unwired: 4 in]
        n171 = call "PADMINI_AUTO_CYCLE VALUE 50.vi"("Enum"=enum16{"Read", "Write"}."Write", "error in (no error)"=w515, "Input"=w513) -> ("error out"=w514:errorcluster)  [unwired: 7 in, 1 out]
        n172 = call-poly <vilib>:"read DB.vi"("Item offset [byte]"=u32 20, "String length reserved in DB (default=254)"=u16 50, "error in (no error)"=w514, "items #"=u16 1 ("Items # [byte]"), "Data Block #"=w501, "S7 Connection in"=w521) -> ("error out"=w504:errorcluster, "STRING result Array"=w500:string[], "S7 Connection out"=w503:T4)  [unwired: 2 in, 1 out]
        n173 = call-poly <vilib>:"read DB.vi"("Item offset [byte]"=u32 72, "String length reserved in DB (default=254)"=u16 10, "error in (no error)"=w504, "items #"=u16 5 ("Items # [byte]"), "Data Block #"=w501, "S7 Connection in"=w503) -> ("error out"=w505:errorcluster, "STRING result Array"=w499:string[], "S7 Connection out"=w502:T4)  [unwired: 2 in, 1 out]
        n174 = Build Array (concatenate)(w500, w499) -> (w498:string[])
        n175 = call "PADMINI_AUTO_BARCODE_STRING 50.vi"("Enum"=enum16{"Read", "Write"}."Write", "error in (no error)"=w505, "Input"=w498) -> ("error out"=w512:errorcluster)  [unwired: 7 in, 1 out]
      }
      frame #1 {
        # "RECONNECT"
        n176 = case shown="Error" w560 {
          selector: w560 -> [w565 w573]
          tunnel: [w564 w570] -> w558
          tunnel: [w565 w571] -> w559
          tunnel: w561 -> [w564 w567]
          tunnel: w557 -> [_ w566]
          frame No Error {
          }
          frame Error {
            n177 = call <vilib>:"Clear Errors.vi"("error in (no error)"=w573) -> ("error out"=w574:errorcluster)  [unwired: 5 in, 1 out]
            n178 = call <vilib>:"disconnect.vi"("error in (no error)"=w574, "S7 Connection in"=w567) -> ("error out"=w572:errorcluster)  [unwired: 8 in, 1 out]
            n179 = call <vilib>:"Clear Errors.vi"("error in (no error)"=w572) -> ("error out"=w569:errorcluster)  [unwired: 5 in, 1 out]
            n180 = call <vilib>:"connect.vi"("PLC Type"=PLC_Type."S7 1200" ("PLC Type 2"), "error in (no error)"=w569, "IP address"=w566) -> ("error out"=w571:errorcluster, "S7 Connection out"=w570:T4)  [unwired: 7 in]
          }
        }
        n181 = Unbundle By Name(w560) -> ("status"=w563:bool)
        n182 = Not(x=w563) -> (.not. x?=w562:bool)
        "PLC 4" <- w562
        n183 = global write "Global 1.vi" "PLC 4"(w562) -> ()
      }
    }
    n184 = call "PADMINI_STOP_ALL.vi"("Enum"=enum16{"Read", "Write"}."Read") -> ("Boolean 2"=w475:bool)  [unwired: 9 in, 1 out]
    n185 = local read "stop"() -> (w474:bool)
    n186 = Or(x=w474, y=w475) -> (x .or. y?=w473:bool)
    n187 = Wait (ms)(milliseconds to wait=u32 50) -> ()  [unwired: 1 out]
  }
  n188 = while {
    shift-right: [w577] -> w52
    shift-left: w55 -> [w587]
    shift-right: [w585] -> w53
    shift-left: w56 -> [w586]
    tunnel: w28 -> [w576]
    stop <- w579 stop-if-true
    # "OP 70 - 80"
    n189 = flat-sequence {
      tunnel: [w598] -> w583
      tunnel: [w646] -> w578
      tunnel: w586 -> [w684]
      tunnel: w587 -> [w683]
      tunnel: w576 -> [w665]
      tunnel: [w665] -> w575
      tunnel: [w737] -> w585
      tunnel: [w736] -> w577
      tunnel: w583 -> [w739]
      tunnel: w578 -> [w738]
      tunnel: w575 -> [w735]
      frame #0 {
        w614 = u16 83 ("Data Block #")
        w639 = u16 81 ("Data Block #")
        w597 = u16 82 ("Data Block #")
        w620 = u16 80 ("Data Block #")
        # "AUTO WRITE"
        n190 = global read "DATA LOG.vi" "OP 70 Outputs"() -> (w682:bool)
        n191 = case shown="True" w682 {
          tunnel: w683 -> [w720 w733]
          tunnel: [w721 w724] -> w644
          tunnel: [w720 w725] -> w643
          tunnel: w684 -> [w721 w730]
          frame False {
          }
          frame True {
            w734 = u16 81  # Data Block #
            n192 = call "PADMINI_AUTO_BARCODE_STATUS 70.vi"("Enum"=enum16{"Read", "Write"}."Read", "error in (no error)"=w730) -> ("error out"=w729:errorcluster, "O/P"=w731:i32[])  [unwired: 8 in]
            n193 = global write "DATA LOG.vi" "OP 70 Outputs"(FALSE) -> ()
            n194 = call-poly <vilib>:"write DB.vi"("DINT input array"=w731, "error in (no error)"=w729, "Data Block #"=w734, "S7 Connection in"=w733) -> ("error out"=w722:errorcluster, "S7 Connection out"=w723:T4)  [unwired: 4 in, 2 out]
            n195 = call-poly <vilib>:"write DB.vi"("DINT input array"=i32[] [0] ("Data Byte"), "error in (no error)"=w722, "Data Block #"=u16 80, "S7 Connection in"=w723) -> ("error out"=w724:errorcluster, "S7 Connection out"=w725:T4)  [unwired: 4 in, 2 out]
          }
        }
        n196 = global read "DATA LOG.vi" "OP 70 reset"() -> (w645:bool)
        n197 = global read "DATA LOG.vi" "Auto Cycle On"() -> (w590:bool)
        n198 = case shown="True" w645 {
          tunnel: w644 -> [w695 w704]
          tunnel: [w695 w703] -> w634
          tunnel: w643 -> [w696 w702]
          tunnel: [w696 w701] -> w635
          frame False {
          }
          frame True {
            n199 = global write "DATA LOG.vi" "OP 70 reset"(FALSE) -> ()
            n200 = call-poly <vilib>:"write DB.vi"("Item offset [byte]"=u16 4 ("Data Block #"), "DINT input array"=i32[] [0], "error in (no error)"=w704, "Data Block #"=u16 80, "S7 Connection in"=w702) -> ("error out"=w703:errorcluster, "S7 Connection out"=w701:T4)  [unwired: 3 in, 2 out]
          }
        }
        n201 = Boolean To (0,1)(Boolean=w590) -> (0, 1=w589:i16)
        n202 = Build Array(w589) -> (w588:i16[])
        n203 = global read "Global 1.vi" "Filtered BARCODE selected"() -> (w636:string[])
        n204 = call-poly <vilib>:"write DB.vi"("Item offset [byte]"=u32 20, "DINT input array"=w588, "error in (no error)"=w634, "Data Block #"=w639, "S7 Connection in"=w635) -> ("error out"=w641:errorcluster, "S7 Connection out"=w642:T4)  [unwired: 3 in, 2 out]
        n205 = call-poly <vilib>:"write DB.vi"("Item offset [byte]"=u32 24, "Input STRINGS"=w636, "error in (no error)"=w641, "String length reserved in DB (default=254)"=u16 15, "Data Block #"=w639, "S7 Connection in"=w642) -> ("error out"=w632:errorcluster, "S7 Connection out"=w633:T4)  [unwired: 2 in, 2 out]
        n206 = call-poly <vilib>:"read DB.vi"("error in (no error)"=w632, "items #"=u16 2 ("Items # [byte]"), "Data Block #"=w620, "S7 Connection in"=w633) -> ("error out"=w680:errorcluster, "DINT result array"=w678:i32[], "S7 Connection out"=w675:T4)  [unwired: 5 in]
        n207 = call "PADMINI_AUTO_CYCLE STATE 70.vi"("Enum"=enum16{"Read", "Write"}."Write", "error in (no error)"=w680, "Input"=w678) -> ("error out"=w676:errorcluster)  [unwired: 7 in, 1 out]
        n208 = call-poly <vilib>:"read DB.vi"("Item offset [byte]"=u32 8, "error in (no error)"=w676, "items #"=u16 2 ("Items # [byte]"), "Data Block #"=w620, "S7 Connection in"=w675) -> ("error out"=w668:errorcluster, "REAL result array"=w666:sgl[], "S7 Connection out"=w674:T4)  [unwired: 4 in]
        n209 = call "PADMINI_AUTO_CYCLE VALUE 70.vi"("Enum"=enum16{"Read", "Write"}."Write", "error in (no error)"=w668, "Input"=w666) -> ("error out"=w667:errorcluster)  [unwired: 7 in, 1 out]
        n210 = call-poly <vilib>:"read DB.vi"("Item offset [byte]"=u32 16, "String length reserved in DB (default=254)"=u16 50, "error in (no error)"=w667, "items #"=u16 1 ("Items # [byte]"), "Data Block #"=w620, "S7 Connection in"=w674) -> ("error out"=w625:errorcluster, "STRING result Array"=w624:string[], "S7 Connection out"=w626:T4)  [unwired: 2 in, 1 out]
        n211 = call-poly <vilib>:"read DB.vi"("Item offset [byte]"=u32 68, "String length reserved in DB (default=254)"=u16 10, "error in (no error)"=w625, "items #"=u16 1 ("Items # [byte]"), "Data Block #"=w620, "S7 Connection in"=w626) -> ("error out"=w627:errorcluster, "STRING result Array"=w628:string[], "S7 Connection out"=w621:T4)  [unwired: 2 in, 1 out]
        n212 = Build Array (concatenate)(w624, w628) -> (w622:string[])
        n213 = call "PADMINI_AUTO_BARCODE_STRING 70.vi"("Enum"=enum16{"Read", "Write"}."Write", "error in (no error)"=w627, "Input"=w622) -> ("error out"=w647:errorcluster)  [unwired: 7 in, 1 out]
        n214 = global read "DATA LOG.vi" "OP 80 Outputs"() -> (w648:bool)
        n215 = case shown="True" w648 {
          tunnel: [w706 w709] -> w619
          tunnel: [w705 w710] -> w595
          tunnel: w647 -> [w706 w716]
          tunnel: w621 -> [w705 w713]
          frame False {
          }
          frame True {
            w719 = u16 83  # Data Block #
            n216 = call "PADMINI_AUTO_BARCODE_STATUS 80.vi"("Enum"=enum16{"Read", "Write"}."Read", "error in (no error)"=w716) -> ("error out"=w715:errorcluster, "O/P"=w717:i32[])  [unwired: 8 in]
            n217 = global write "DATA LOG.vi" "OP 80 Outputs"(FALSE) -> ()
            n218 = call-poly <vilib>:"write DB.vi"("DINT input array"=w717, "error in (no error)"=w715, "Data Block #"=w719, "S7 Connection in"=w713) -> ("error out"=w707:errorcluster, "S7 Connection out"=w708:T4)  [unwired: 4 in, 2 out]
            n219 = call-poly <vilib>:"write DB.vi"("DINT input array"=i32[] [0] ("Data Byte"), "error in (no error)"=w707, "Data Block #"=u16 82, "S7 Connection in"=w708) -> ("error out"=w709:errorcluster, "S7 Connection out"=w710:T4)  [unwired: 4 in, 2 out]
          }
        }
        n220 = global read "DATA LOG.vi" "OP 80 reset"() -> (w618:bool)
        n221 = global read "DATA LOG.vi" "Auto Cycle On"() -> (w593:bool)
        n222 = case shown="True" w618 {
          tunnel: w619 -> [w686 w694]
          tunnel: [w686 w689] -> _
          tunnel: [w686 w689] -> w608
          tunnel: w595 -> [w685 w688]
          tunnel: [w685 w687] -> w594
          frame False {
          }
          frame True {
            n223 = global write "DATA LOG.vi" "OP 80 reset"(FALSE) -> ()
            n224 = call-poly <vilib>:"write DB.vi"("Item offset [byte]"=u16 4 ("Data Block #"), "DINT input array"=i32[] [0], "error in (no error)"=w694, "Data Block #"=u16 82, "S7 Connection in"=w688) -> ("error out"=w689:errorcluster, "S7 Connection out"=w687:T4)  [unwired: 3 in, 2 out]
          }
        }
        n225 = Boolean To (0,1)(Boolean=w593) -> (0, 1=w592:i16)
        n226 = Build Array(w592) -> (w591:i16[])
        n227 = global read "Global 1.vi" "Filtered BARCODE selected"() -> (w611:string[])
        n228 = call-poly <vilib>:"write DB.vi"("Item offset [byte]"=u32 20, "DINT input array"=w591, "error in (no error)"=w608, "Data Block #"=w614, "S7 Connection in"=w594) -> ("error out"=w616:errorcluster, "S7 Connection out"=w617:T4)  [unwired: 3 in, 2 out]
        n229 = call-poly <vilib>:"write DB.vi"("Item offset [byte]"=u32 24, "Input STRINGS"=w611, "error in (no error)"=w616, "String length reserved in DB (default=254)"=u16 15, "Data Block #"=w614, "S7 Connection in"=w617) -> ("error out"=w609:errorcluster, "S7 Connection out"=w610:T4)  [unwired: 2 in, 2 out]
        n230 = call-poly <vilib>:"read DB.vi"("error in (no error)"=w609, "items #"=u16 2 ("Items # [byte]"), "Data Block #"=w597, "S7 Connection in"=w610) -> ("error out"=w650:errorcluster, "DINT result array"=w652:i32[], "S7 Connection out"=w655:T4)  [unwired: 5 in]
        n231 = call "PADMINI_AUTO_CYCLE STATE 80.vi"("Enum"=enum16{"Read", "Write"}."Write", "error in (no error)"=w650, "Input"=w652) -> ("error out"=w654:errorcluster)  [unwired: 7 in, 1 out]
        n232 = call-poly <vilib>:"read DB.vi"("Item offset [byte]"=u32 8, "error in (no error)"=w654, "items #"=u16 1 ("Items # [byte]"), "Data Block #"=w597, "S7 Connection in"=w655) -> ("error out"=w662:errorcluster, "REAL result array"=w664:sgl[], "S7 Connection out"=w656:T4)  [unwired: 4 in]
        n233 = call "PADMINI_AUTO_CYCLE VALUE 80.vi"("Enum"=enum16{"Read", "Write"}."Write", "error in (no error)"=w662, "Input"=w664) -> ("error out"=w663:errorcluster)  [unwired: 7 in, 1 out]
        n234 = call-poly <vilib>:"read DB.vi"("Item offset [byte]"=u32 12, "String length reserved in DB (default=254)"=u16 50, "error in (no error)"=w663, "items #"=u16 1 ("Items # [byte]"), "Data Block #"=w597, "S7 Connection in"=w656) -> ("error out"=w603:errorcluster, "STRING result Array"=w601:string[], "S7 Connection out"=w599:T4)  [unwired: 2 in, 1 out]
        n235 = call-poly <vilib>:"read DB.vi"("Item offset [byte]"=u32 64, "String length reserved in DB (default=254)"=u16 10, "error in (no error)"=w603, "items #"=u16 2 ("Items # [byte]"), "Data Block #"=w597, "S7 Connection in"=w599) -> ("error out"=w602:errorcluster, "STRING result Array"=w607:string[], "S7 Connection out"=w598:T4)  [unwired: 2 in, 1 out]
        n236 = Build Array (concatenate)(w601, w607) -> (w600:string[])
        n237 = call "PADMINI_AUTO_BARCODE_STRING 80.vi"("Enum"=enum16{"Read", "Write"}."Write", "error in (no error)"=w602, "Input"=w600) -> ("error out"=w646:errorcluster)  [unwired: 7 in, 1 out]
      }
      frame #1 {
        # "RECONNECT"
        n238 = case shown="Error" w738 {
          selector: w738 -> [w743 w751]
          tunnel: [w742 w748] -> w736
          tunnel: [w743 w749] -> w737
          tunnel: w739 -> [w742 w745]
          tunnel: w735 -> [_ w744]
          frame No Error {
          }
          frame Error {
            n239 = call <vilib>:"Clear Errors.vi"("error in (no error)"=w751) -> ("error out"=w752:errorcluster)  [unwired: 5 in, 1 out]
            n240 = call <vilib>:"disconnect.vi"("error in (no error)"=w752, "S7 Connection in"=w745) -> ("error out"=w750:errorcluster)  [unwired: 8 in, 1 out]
            n241 = call <vilib>:"Clear Errors.vi"("error in (no error)"=w750) -> ("error out"=w747:errorcluster)  [unwired: 5 in, 1 out]
            n242 = call <vilib>:"connect.vi"("PLC Type"=PLC_Type."S7 1200" ("PLC Type 2"), "error in (no error)"=w747, "IP address"=w744) -> ("error out"=w749:errorcluster, "S7 Connection out"=w748:T4)  [unwired: 7 in]
          }
        }
        n243 = Unbundle By Name(w738) -> ("status"=w741:bool)
        n244 = Not(x=w741) -> (.not. x?=w740:bool)
        "PLC 6" <- w740
        n245 = global write "Global 1.vi" "PLC 6"(w740) -> ()
      }
    }
    n246 = call "PADMINI_STOP_ALL.vi"("Enum"=enum16{"Read", "Write"}."Read") -> ("Boolean 2"=w581:bool)  [unwired: 9 in, 1 out]
    n247 = local read "stop"() -> (w580:bool)
    n248 = Or(x=w580, y=w581) -> (x .or. y?=w579:bool)
    n249 = Wait (ms)(milliseconds to wait=u32 50) -> ()  [unwired: 1 out]
  }
  n250 = while {
    shift-right: [w755] -> w72
    shift-left: w75 -> [w765]
    shift-right: [w763] -> w73
    shift-left: w76 -> [w764]
    tunnel: w71 -> [w754]
    stop <- w757 stop-if-true
    # "OP 60"
    n251 = flat-sequence {
      tunnel: [w774] -> w761
      tunnel: [w796] -> w756
      tunnel: w764 -> [w815]
      tunnel: w765 -> [w814]
      tunnel: w754 -> [w795]
      tunnel: [w795] -> w753
      tunnel: [w843] -> w763
      tunnel: [w842] -> w755
      tunnel: w761 -> [w845]
      tunnel: w756 -> [w844]
      tunnel: w753 -> [w841]
      frame #0 {
        w791 = u16 44 ("Data Block #")
        w771 = u16 43 ("Data Block #")
        # "AUTO WRITE"
        n252 = global read "DATA LOG.vi" "OP 60 Outputs"() -> (w813:bool)
        n253 = case shown="True" w813 {
          tunnel: w814 -> [w826 w839]
          tunnel: [w827 w828] -> w783
          tunnel: [w826 w831] -> w782
          tunnel: w815 -> [w827 w836]
          frame False {
          }
          frame True {
            w840 = u16 44  # Data Block #
            n254 = call "PADMINI_AUTO_BARCODE_STATUS 60.vi"("Enum"=enum16{"Read", "Write"}."Read", "error in (no error)"=w836) -> ("error out"=w835:errorcluster, "O/P"=w837:i32[])  [unwired: 8 in]
            n255 = global write "DATA LOG.vi" "OP 60 Outputs"(FALSE) -> ()
            n256 = call-poly <vilib>:"write DB.vi"("DINT input array"=w837, "error in (no error)"=w835, "Data Block #"=w840, "S7 Connection in"=w839) -> ("error out"=w829:errorcluster, "S7 Connection out"=w830:T4)  [unwired: 4 in, 2 out]
            n257 = call-poly <vilib>:"write DB.vi"("DINT input array"=i32[] [0] ("Data Byte"), "error in (no error)"=w829, "Data Block #"=u16 43, "S7 Connection in"=w830) -> ("error out"=w828:errorcluster, "S7 Connection out"=w831:T4)  [unwired: 4 in, 2 out]
          }
        }
        n258 = global read "DATA LOG.vi" "OP 60 reset"() -> (w781:bool)
        n259 = global read "DATA LOG.vi" "Auto Cycle On"() -> (w768:bool)
        n260 = case shown="True" w781 {
          tunnel: w783 -> [w816 w825]
          tunnel: [w816 w824] -> w784
          tunnel: w782 -> [w817 w823]
          tunnel: [w817 w822] -> w785
          frame False {
          }
          frame True {
            n261 = global write "DATA LOG.vi" "OP 60 reset"(FALSE) -> ()
            n262 = call-poly <vilib>:"write DB.vi"("Item offset [byte]"=u16 4 ("Data Block #"), "DINT input array"=i32[] [0], "error in (no error)"=w825, "Data Block #"=u16 43, "S7 Connection in"=w823) -> ("error out"=w824:errorcluster, "S7 Connection out"=w822:T4)  [unwired: 3 in, 2 out]
          }
        }
        n263 = Boolean To (0,1)(Boolean=w768) -> (0, 1=w767:i16)
        n264 = Build Array(w767) -> (w766:i16[])
        n265 = global read "Global 1.vi" "Filtered BARCODE selected"() -> (w794:string[])
        n266 = call-poly <vilib>:"write DB.vi"("Item offset [byte]"=u32 20, "DINT input array"=w766, "error in (no error)"=w784, "Data Block #"=w791, "S7 Connection in"=w785) -> ("error out"=w789:errorcluster, "S7 Connection out"=w788:T4)  [unwired: 3 in, 2 out]
        n267 = call-poly <vilib>:"write DB.vi"("Item offset [byte]"=u32 24, "Input STRINGS"=w794, "error in (no error)"=w789, "String length reserved in DB (default=254)"=u16 15, "Data Block #"=w791, "S7 Connection in"=w788) -> ("error out"=w786:errorcluster, "S7 Connection out"=w787:T4)  [unwired: 2 in, 2 out]
        n268 = call-poly <vilib>:"read DB.vi"("error in (no error)"=w786, "items #"=u16 2 ("Items # [byte]"), "Data Block #"=w771, "S7 Connection in"=w787) -> ("error out"=w811:errorcluster, "DINT result array"=w809:i32[], "S7 Connection out"=w806:T4)  [unwired: 5 in]
        n269 = call "PADMINI_AUTO_CYCLE STATE 60.vi"("Enum"=enum16{"Read", "Write"}."Write", "error in (no error)"=w811, "Input"=w809) -> ("error out"=w807:errorcluster)  [unwired: 7 in, 1 out]
        n270 = call-poly <vilib>:"read DB.vi"("Item offset [byte]"=u32 8, "error in (no error)"=w807, "items #"=u16 6 ("Items # [byte]"), "Data Block #"=w771, "S7 Connection in"=w806) -> ("error out"=w799:errorcluster, "REAL result array"=w797:sgl[], "S7 Connection out"=w805:T4)  [unwired: 4 in]
        n271 = call "PADMINI_AUTO_CYCLE VALUE 60.vi"("Enum"=enum16{"Read", "Write"}."Write", "error in (no error)"=w799, "Input"=w797) -> ("error out"=w798:errorcluster)  [unwired: 7 in, 1 out]
        n272 = call-poly <vilib>:"read DB.vi"("Item offset [byte]"=u32 32, "String length reserved in DB (default=254)"=u16 50, "error in (no error)"=w798, "items #"=u16 1 ("Items # [byte]"), "Data Block #"=w771, "S7 Connection in"=w805) -> ("error out"=w776:errorcluster, "STRING result Array"=w773:string[], "S7 Connection out"=w775:T4)  [unwired: 2 in, 1 out]
        n273 = call-poly <vilib>:"read DB.vi"("Item offset [byte]"=u32 84, "String length reserved in DB (default=254)"=u16 10, "error in (no error)"=w776, "items #"=u16 7 ("Items # [byte]"), "Data Block #"=w771, "S7 Connection in"=w775) -> ("error out"=w777:errorcluster, "STRING result Array"=w780:string[], "S7 Connection out"=w774:T4)  [unwired: 2 in, 1 out]
        n274 = Build Array (concatenate)(w773, w780) -> (w772:string[])
        n275 = call "PADMINI_AUTO_BARCODE_STRING 60.vi"("Enum"=enum16{"Read", "Write"}."Write", "error in (no error)"=w777, "Input"=w772) -> ("error out"=w796:errorcluster)  [unwired: 7 in, 1 out]
      }
      frame #1 {
        # "RECONNECT"
        n276 = case shown="Error" w844 {
          selector: w844 -> [w849 w857]
          tunnel: [w848 w854] -> w842
          tunnel: [w849 w855] -> w843
          tunnel: w845 -> [w848 w851]
          tunnel: w841 -> [_ w850]
          frame No Error {
          }
          frame Error {
            n277 = call <vilib>:"Clear Errors.vi"("error in (no error)"=w857) -> ("error out"=w858:errorcluster)  [unwired: 5 in, 1 out]
            n278 = call <vilib>:"disconnect.vi"("error in (no error)"=w858, "S7 Connection in"=w851) -> ("error out"=w856:errorcluster)  [unwired: 8 in, 1 out]
            n279 = call <vilib>:"Clear Errors.vi"("error in (no error)"=w856) -> ("error out"=w853:errorcluster)  [unwired: 5 in, 1 out]
            n280 = call <vilib>:"connect.vi"("PLC Type"=PLC_Type."S7 1200" ("PLC Type 2"), "error in (no error)"=w853, "IP address"=w850) -> ("error out"=w855:errorcluster, "S7 Connection out"=w854:T4)  [unwired: 7 in]
          }
        }
        n281 = Unbundle By Name(w844) -> ("status"=w847:bool)
        n282 = Not(x=w847) -> (.not. x?=w846:bool)
        "PLC 5" <- w846
        n283 = global write "Global 1.vi" "PLC 5"(w846) -> ()
      }
    }
    n284 = call "PADMINI_STOP_ALL.vi"("Enum"=enum16{"Read", "Write"}."Read") -> ("Boolean 2"=w759:bool)  [unwired: 9 in, 1 out]
    n285 = local read "stop"() -> (w758:bool)
    n286 = Or(x=w758, y=w759) -> (x .or. y?=w757:bool)
    n287 = Wait (ms)(milliseconds to wait=u32 50) -> ()  [unwired: 1 out]
  }
  n288 = while {
    shift-right: [w861] -> w107
    shift-left: w111 -> [w871]
    shift-right: [w869] -> w108
    shift-left: w112 -> [w870]
    tunnel: w110 -> [w860]
    stop <- w863 stop-if-true
    # "OP 40"
    n289 = flat-sequence {
      tunnel: [w883] -> w867
      tunnel: [w902] -> w862
      tunnel: w870 -> [w921]
      tunnel: w871 -> [w920]
      tunnel: w860 -> [w901]
      tunnel: [w901] -> w859
      tunnel: [w949] -> w869
      tunnel: [w948] -> w861
      tunnel: w867 -> [w951]
      tunnel: w862 -> [w950]
      tunnel: w859 -> [w947]
      frame #0 {
        w894 = u16 57 ("Data Block #")
        w882 = u16 56 ("Data Block #")
        # "AUTO WRITE"
        n290 = global read "DATA LOG.vi" "OP 40 Outputs"() -> (w919:bool)
        n291 = case shown="True" w919 {
          tunnel: w920 -> [w932 w945]
          tunnel: [w933 w937] -> w899
          tunnel: [w932 w939] -> w900
          tunnel: w921 -> [w933 w942]
          frame False {
          }
          frame True {
            w946 = u16 57  # Data Block #
            n292 = call "PADMINI_AUTO_BARCODE_STATUS 40.vi"("Enum"=enum16{"Read", "Write"}."Read", "error in (no error)"=w942) -> ("error out"=w941:errorcluster, "O/P"=w943:i32[])  [unwired: 8 in]
            n293 = global write "DATA LOG.vi" "OP 40 Outputs"(FALSE) -> ()
            n294 = call-poly <vilib>:"write DB.vi"("DINT input array"=w943, "error in (no error)"=w941, "Data Block #"=w946, "S7 Connection in"=w945) -> ("error out"=w936:errorcluster, "S7 Connection out"=w938:T4)  [unwired: 4 in, 2 out]
            n295 = call-poly <vilib>:"write DB.vi"("DINT input array"=i32[] [0], "error in (no error)"=w936, "Data Block #"=u16 56, "S7 Connection in"=w938) -> ("error out"=w937:errorcluster, "S7 Connection out"=w939:T4)  [unwired: 4 in, 2 out]
          }
        }
        n296 = global read "DATA LOG.vi" "OP 40 reset"() -> (w898:bool)
        n297 = global read "DATA LOG.vi" "Auto Cycle On"() -> (w874:bool)
        n298 = case shown="True" w898 {
          tunnel: w899 -> [w922 w931]
          tunnel: [w922 w930] -> w887
          tunnel: w900 -> [w923 w929]
          tunnel: [w923 w928] -> w888
          frame False {
          }
          frame True {
            n299 = global write "DATA LOG.vi" "OP 40 reset"(FALSE) -> ()
            n300 = call-poly <vilib>:"write DB.vi"("Item offset [byte]"=u16 4 ("Data Block #"), "DINT input array"=i32[] [0], "error in (no error)"=w931, "Data Block #"=u16 56, "S7 Connection in"=w929) -> ("error out"=w930:errorcluster, "S7 Connection out"=w928:T4)  [unwired: 3 in, 2 out]
          }
        }
        n301 = Boolean To (0,1)(Boolean=w874) -> (0, 1=w873:i16)
        n302 = Build Array(w873) -> (w872:i16[])
        n303 = global read "Global 1.vi" "Filtered BARCODE selected"() -> (w897:string[])
        n304 = call-poly <vilib>:"write DB.vi"("Item offset [byte]"=u32 20, "DINT input array"=w872, "error in (no error)"=w887, "Data Block #"=w894, "S7 Connection in"=w888) -> ("error out"=w892:errorcluster, "S7 Connection out"=w891:T4)  [unwired: 3 in, 2 out]
        n305 = call-poly <vilib>:"write DB.vi"("Item offset [byte]"=u32 24, "Input STRINGS"=w897, "error in (no error)"=w892, "String length reserved in DB (default=254)"=u16 15, "Data Block #"=w894, "S7 Connection in"=w891) -> ("error out"=w889:errorcluster, "S7 Connection out"=w890:T4)  [unwired: 2 in, 2 out]
        n306 = call-poly <vilib>:"read DB.vi"("error in (no error)"=w889, "items #"=u16 2 ("Items # [byte]"), "Data Block #"=w882, "S7 Connection in"=w890) -> ("error out"=w917:errorcluster, "DINT result array"=w915:i32[], "S7 Connection out"=w912:T4)  [unwired: 5 in]
        n307 = call "PADMINI_AUTO_CYCLE STATE 40.vi"("Enum"=enum16{"Read", "Write"}."Write", "error in (no error)"=w917, "Input"=w915) -> ("error out"=w913:errorcluster)  [unwired: 7 in, 1 out]
        n308 = call-poly <vilib>:"read DB.vi"("Item offset [byte]"=u32 8, "error in (no error)"=w913, "items #"=u16 4 ("Items # [byte]"), "Data Block #"=w882, "S7 Connection in"=w912) -> ("error out"=w905:errorcluster, "REAL result array"=w903:sgl[], "S7 Connection out"=w911:T4)  [unwired: 4 in]
        n309 = call "PADMINI_AUTO_CYCLE VALUE 40.vi"("Enum"=enum16{"Read", "Write"}."Write", "error in (no error)"=w905, "Input"=w903) -> ("error out"=w904:errorcluster)  [unwired: 7 in, 1 out]
        n310 = call-poly <vilib>:"read DB.vi"("Item offset [byte]"=u32 24, "String length reserved in DB (default=254)"=u16 50, "error in (no error)"=w904, "items #"=u16 1 ("Items # [byte]"), "Data Block #"=w882, "S7 Connection in"=w911) -> ("error out"=w886:errorcluster, "STRING result Array"=w877:string[], "S7 Connection out"=w884:T4)  [unwired: 2 in, 1 out]
        n311 = call-poly <vilib>:"read DB.vi"("Item offset [byte]"=u32 76, "String length reserved in DB (default=254)"=u16 10, "error in (no error)"=w886, "items #"=u16 4 ("Items # [byte]"), "Data Block #"=w882, "S7 Connection in"=w884) -> ("error out"=w885:errorcluster, "STRING result Array"=w876:string[], "S7 Connection out"=w883:T4)  [unwired: 2 in, 1 out]
        n312 = Build Array (concatenate)(w877, w876) -> (w875:string[])
        n313 = call "PADMINI_AUTO_BARCODE_STRING 40.vi"("Enum"=enum16{"Read", "Write"}."Write", "error in (no error)"=w885, "Input"=w875) -> ("error out"=w902:errorcluster)  [unwired: 7 in, 1 out]
      }
      frame #1 {
        # "RECONNECT"
        n314 = case shown="Error" w950 {
          selector: w950 -> [w955 w963]
          tunnel: [w954 w960] -> w948
          tunnel: [w955 w961] -> w949
          tunnel: w951 -> [w954 w957]
          tunnel: w947 -> [_ w956]
          frame No Error {
          }
          frame Error {
            n315 = call <vilib>:"Clear Errors.vi"("error in (no error)"=w963) -> ("error out"=w964:errorcluster)  [unwired: 5 in, 1 out]
            n316 = call <vilib>:"disconnect.vi"("error in (no error)"=w964, "S7 Connection in"=w957) -> ("error out"=w962:errorcluster)  [unwired: 8 in, 1 out]
            n317 = call <vilib>:"Clear Errors.vi"("error in (no error)"=w962) -> ("error out"=w959:errorcluster)  [unwired: 5 in, 1 out]
            n318 = call <vilib>:"connect.vi"("PLC Type"=PLC_Type."S7 1200" ("PLC Type 2"), "error in (no error)"=w959, "IP address"=w956) -> ("error out"=w961:errorcluster, "S7 Connection out"=w960:T4)  [unwired: 7 in]
          }
        }
        n319 = Unbundle By Name(w950) -> ("status"=w953:bool)
        n320 = Not(x=w953) -> (.not. x?=w952:bool)
        "PLC 3" <- w952
        n321 = global write "Global 1.vi" "PLC 3"(w952) -> ()
      }
    }
    n322 = call "PADMINI_STOP_ALL.vi"("Enum"=enum16{"Read", "Write"}."Read") -> ("Boolean 2"=w865:bool)  [unwired: 9 in, 1 out]
    n323 = local read "stop"() -> (w864:bool)
    n324 = Or(x=w864, y=w865) -> (x .or. y?=w863:bool)
    n325 = Wait (ms)(milliseconds to wait=u32 50) -> ()  [unwired: 1 out]
  }
  n326 = call <vilib>:"Clear Errors.vi"("error in (no error)"=w108) -> ("error out"=w109:errorcluster)  [unwired: 5 in, 1 out]
  n327 = call <vilib>:"Clear Errors.vi"("error in (no error)"=w117) -> ("error out"=w119:errorcluster)  [unwired: 5 in, 1 out]
  n328 = call <vilib>:"Clear Errors.vi"("error in (no error)"=w94) -> ("error out"=w93:errorcluster)  [unwired: 5 in, 1 out]
  n329 = call <vilib>:"Clear Errors.vi"("error in (no error)"=w73) -> ("error out"=w74:errorcluster)  [unwired: 5 in, 1 out]
  n330 = call <vilib>:"disconnect.vi"("error in (no error)"=w109, "S7 Connection in"=w107) -> ("error out"=w106:errorcluster)  [unwired: 8 in, 1 out]
  n331 = call <vilib>:"disconnect.vi"("error in (no error)"=w119, "S7 Connection in"=w118) -> ("error out"=w105:errorcluster)  [unwired: 8 in, 1 out]
  n332 = call <vilib>:"disconnect.vi"("error in (no error)"=w93, "S7 Connection in"=w95) -> ("error out"=w70:errorcluster)  [unwired: 8 in, 1 out]
  n333 = call <vilib>:"disconnect.vi"("error in (no error)"=w74, "S7 Connection in"=w72) -> ("error out"=w69:errorcluster)  [unwired: 8 in, 1 out]
  n334 = Merge Errors(w105, w106, w70, w69) -> (w104:errorcluster)
  n335 = call <vilib>:"Clear Errors.vi"("error in (no error)"=w53) -> ("error out"=w54:errorcluster)  [unwired: 5 in, 1 out]
  n336 = call <vilib>:"disconnect.vi"("error in (no error)"=w54, "S7 Connection in"=w52) -> ("error out"=w22:errorcluster)  [unwired: 8 in, 1 out]
  n337 = call <vilib>:"Clear Errors.vi"("error in (no error)"=w160) -> ("error out"=w146:errorcluster)  [unwired: 5 in, 1 out]
  n338 = call <vilib>:"disconnect.vi"("error in (no error)"=w146, "S7 Connection in"=w145) -> ("error out"=w144:errorcluster)  [unwired: 8 in, 1 out]
  n339 = control-ref of="This VI"() -> (w3:refnum<vi>)
  n340 = call <vilib>:"Clear Errors.vi"("error in (no error)"=w24) -> ("error out"=w25:errorcluster)  [unwired: 5 in, 1 out]
  n341 = call <vilib>:"disconnect.vi"("error in (no error)"=w25, "S7 Connection in"=w23) -> ("error out"=w20:errorcluster)  [unwired: 8 in, 1 out]
  n342 = Merge Errors(w22, w20) -> (w21:errorcluster)
  n343 = Merge Errors(w144, w104, w21) -> (w165:errorcluster)
  n344 = call <vilib>:"Simple Error Handler.vi"("type of dialog (OK msg:1)"=w2, "error in (no error)"=w165) -> ("error out"=w164:errorcluster)  [unwired: 3 in, 4 out]
  n345 = call <vilib>:"Clear Errors.vi"("error in (no error)"=w164) -> ("error out"=w163:errorcluster)  [unwired: 5 in, 1 out]
  n346 = invoke class="VI" method="FP.Close"(reference=w3, error in=w163) -> (error out=→"error out":errorcluster)  [unwired: 1 in, 2 out]
